vi "Create Edit Table of Markers.vi"(11 "markers":T1[](array[typedef])) -> (3 "Array":string[](array[string]))   [LabVIEW 2015]
uses:
  MarkersDVRType.ctl
  controls/markerType.ctl
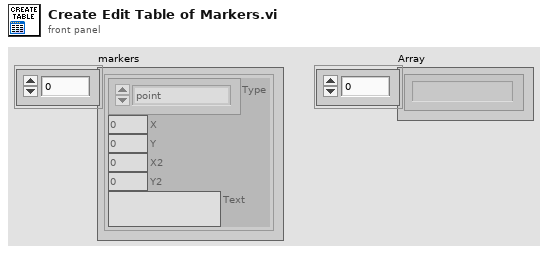
[diagram p1: front panel]
types:
  T1 = typedef "MarkersDVRType.ctl" = cluster{"Type":T2, "X":dbl, "Y":dbl, "X2":dbl, "Y2":dbl, "Text":string}
  T2 = typedef "markerType.ctl" = enum16{"point", "arrow", "horiz", "vert", "vert range", "horiz range", "box"}
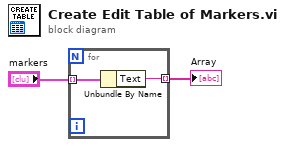
[diagram p0: block diagram]
diagram:
  n1 = for {
    tunnel: "markers" -> [w4] mode=indexing
    tunnel: [w3] -> w1 mode=indexing
    n2 = Unbundle By Name(w4) -> ("Text"=w3:string)
  }
  "Array" <- w1
